vi "Stimulus trigger logic.vi"(7 "Abort triggers":bool, 8 "Unmodified signal values":T2, 9 "Stimulus Trigger Setup":T1={"Trigger period in live protocols (80MHz Cycles)"=80000000, "Pulse width in live protocols (80MHz Cycles)"=40000000, "Enable stimulus in live protocols"=FALSE, "Trigger delay in funct. protocols (80MHz Cycles)"=0, "Pulse width in funct. protocols (80MHz Cycles)"=400000, "Enable stimulus in funct. protocols"=FALSE}, 10 "live_scan":bool, 11 "Imaging Protocol":T3=enum."Live Imaging") -> (1 "Stimulus trigger":bool)   [LabVIEW 2020]
uses:
  <vilib>/eio/EIONode/EIONode.xnode
  <vilib>/rvi/eio/common/nirviEmuTemplateMethod_errors.vi
  Typedefs/Imaging Protocols enum.ctl
  FPGA Typedefs/PXI Trigger lines value cluster.ctl
  FPGA Typedefs/Stimulus trigger delays cluster.ctl
panel:
  # "Limited to 53.5 sec (if U32)"
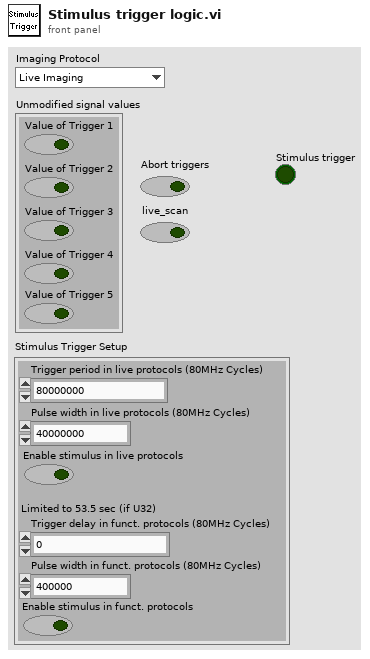
[diagram p1: front panel]
types:
  T1 = typedef "Stimulus trigger delays cluster.ctl" = cluster{"Trigger period in live protocols (80MHz Cycles)":u32, "Pulse width in live protocols (80MHz Cycles)":u32, "Enable stimulus in live protocols":bool, "Trigger delay in funct. protocols (80MHz Cycles)":u32, "Pulse width in funct. protocols (80MHz Cycles)":u32, "Enable stimulus in funct. protocols":bool}
  T2 = typedef "PXI Trigger lines value cluster.ctl" = cluster{"Value of Trigger 1":bool, "Value of Trigger 2":bool, "Value of Trigger 3":bool, "Value of Trigger 4":bool, "Value of Trigger 5":bool}
  T3 = typedef "Imaging Protocols enum.ctl" = enum16{"AOL Z-Stack", "Motor Z Stack", "Functional Acquisition", "Single Plane Acquisition", "Volume Acquisition", "Live Imaging", "Live Plane Imaging", "Live Volume Imaging"}
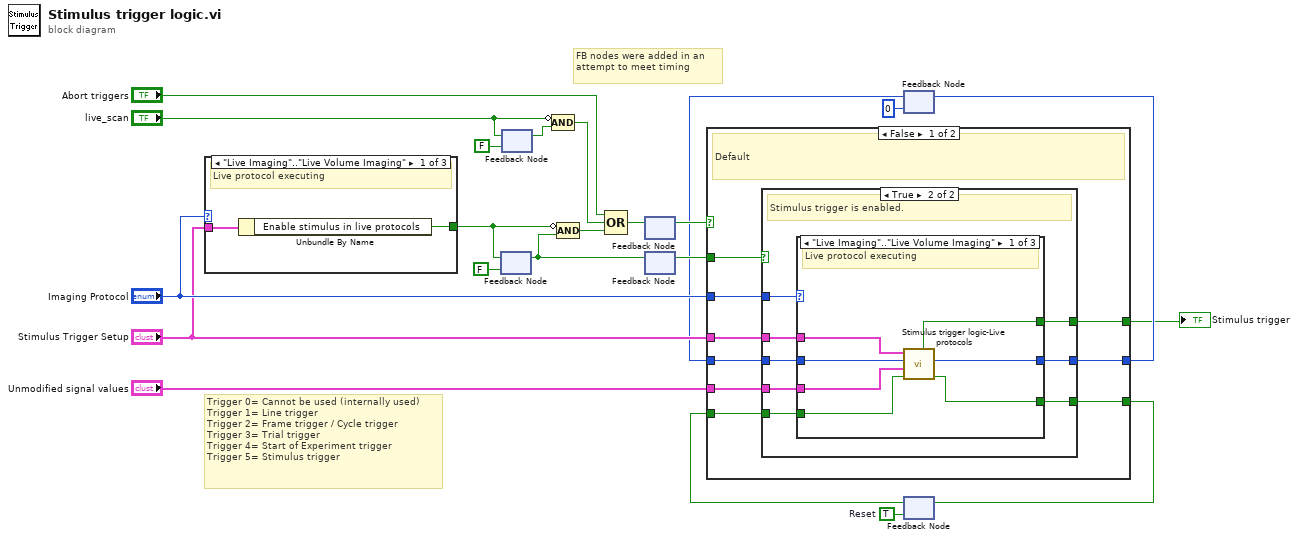
[diagram p0: block diagram]
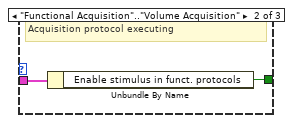
[diagram p2: hidden frame]
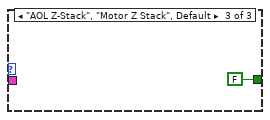
[diagram p3: hidden frame]
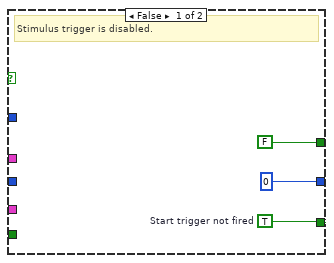
[diagram p4: hidden frame]
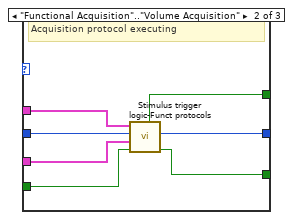
[diagram p5: hidden frame]
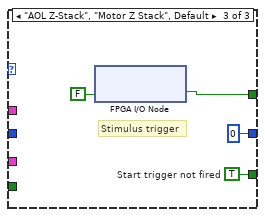
[diagram p6: hidden frame]
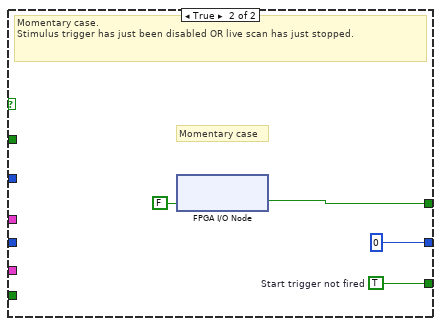
[diagram p7: hidden frame]
diagram:
  w16 = TRUE  # Reset
  # "FB nodes were added in an attempt to meet timing"
  # "Trigger 0= Cannot be used (internally used)\nTrigger 1= Line trigger\nTrigger 2= Frame trigger / Cycle trigger\nTrigger 3= Trial trigger\nTrigger 4= Start of Experiment trigger\nTrigger 5= Stimulus trigger"
  n1 = case shown="\"Live Imaging\"..\"Live Volume Imaging\"" "Imaging Protocol" {
    tunnel: "Stimulus Trigger Setup" -> [w24 w26 _]
    tunnel: [w23 w25 FALSE ("Enable stimulus in live protocols")] -> w12
    frame "Live Imaging".."Live Volume Imaging" {
      # "Live protocol executing"
      n2 = Unbundle By Name(w24) -> ("Enable stimulus in live protocols"=w23:bool)
    }
    frame "Functional Acquisition".."Volume Acquisition" {
      # "Acquisition protocol executing"
      n3 = Unbundle By Name(w26) -> ("Enable stimulus in funct. protocols"=w25:bool)
    }
    frame "AOL Z-Stack", "Motor Z Stack", Default {
    }
  }
  n4 = feedback #1(FALSE ("Trigger 1")) -> (w21:bool)
  n5 = feedback-in #1(w12) -> ()
  n6 = feedback #2(FALSE ("Trigger 1")) -> (w10:bool)
  n7 = feedback-in #2("live_scan") -> ()
  n8 = Compound Arithmetic op=AND(invert "live_scan", w10) -> (w8:bool)
  n9 = Compound Arithmetic op=AND(invert w12, w21) -> (w7:bool)
  n10 = Compound Arithmetic op=OR("Abort triggers", w8, w7) -> (w6:bool)
  n11 = feedback-in #3(w6) -> ()
  n12 = feedback #3() -> (w4:bool)  [unwired: 1 in]
  n13 = feedback-in #4(w21) -> ()
  n14 = feedback #4() -> (w5:bool)  [unwired: 1 in]
  n15 = feedback #5(u32 0 ("Tick Count(Ticks) out")) -> (w2:u32)
  n16 = feedback #6(w16) -> (w3:bool)
  n17 = case shown="False" w4 {
    tunnel: "Imaging Protocol" -> [w36 _]
    tunnel: w5 -> [w35 _]
    tunnel: "Unmodified signal values" -> [w34 _]
    tunnel: "Stimulus Trigger Setup" -> [w33 _]
    tunnel: [w32 w67] -> w18
    tunnel: w3 -> [w31 _]
    tunnel: [w30 u32 0 ("Tick Count(Ticks) out")] -> w19
    tunnel: w2 -> [w29 _]
    tunnel: [w28 w65] -> w15
    frame False {
      # "Default"
      n18 = case shown="True" w35 {
        tunnel: w36 -> [_ w47]
        tunnel: w34 -> [_ w46]
        tunnel: w33 -> [_ w45]
        tunnel: [w39 w41] -> w32
        tunnel: w31 -> [_ w44]
        tunnel: [u32 0 ("Tick Count(Ticks) out") w43] -> w30
        tunnel: w29 -> [_ w42]
        tunnel: [FALSE ("PXI_Trig0") w40] -> w28
        frame False {
          w39 = TRUE  # Start trigger not fired
          # "Stimulus trigger is disabled."
        }
        frame True {
          # "Stimulus trigger is enabled."
          n19 = case shown="\"Live Imaging\"..\"Live Volume Imaging\"" w47 {
            tunnel: w46 -> [w54 w61 _]
            tunnel: w45 -> [w52 w59 _]
            tunnel: w44 -> [w50 w57 _]
            tunnel: [w49 w56 u32 0 ("Tick Count(Ticks) out")] -> w43
            tunnel: w42 -> [w53 w60 _]
            tunnel: [w51 w58 w63] -> w41
            tunnel: [w48 w55 w62] -> w40
            frame "Live Imaging".."Live Volume Imaging" {
              # "Live protocol executing"
              n20 = call "Stimulus trigger logic-Live protocols.vi"("Start trigger not fired"=w50, "Trigger lines value"=w54, "Tick Count(Ticks) in"=w53, "Trigger delays"=w52) -> ("Start trigger not fired"=w51:bool, "Tick Count(Ticks) out"=w49:u32, "Output value"=w48:bool)  [unwired: 5 in]
            }
            frame "Functional Acquisition".."Volume Acquisition" {
              # "Acquisition protocol executing"
              n21 = call "Stimulus trigger logic-Funct protocols.vi"("Start trigger not fired"=w57, "Trigger lines value"=w61, "Tick Count(Ticks) in"=w60, "Stimulus Trigger Setup"=w59) -> ("Start trigger not fired"=w58:bool, "Tick Count(Ticks) out"=w56:u32, "Output value"=w55:bool)  [unwired: 5 in]
            }
            frame "AOL Z-Stack", "Motor Z Stack", Default {
              w62 = FALSE ("PXI_Trig0")
              w63 = TRUE  # Start trigger not fired
              # "Stimulus trigger"
              n22 = xnode "FPGA I/O Node"("PXI_Trig5"=w62) -> ()  [unwired: 1 in, 1 out]
            }
          }
        }
      }
    }
    frame True {
      w65 = FALSE ("PXI_Trig0")
      w67 = TRUE  # Start trigger not fired
      # "Momentary case"
      # "Momentary case.\nStimulus trigger has just been disabled OR live scan has just stopped."
      n23 = xnode "FPGA I/O Node"("PXI_Trig5"=w65) -> ()  [unwired: 1 in, 1 out]
    }
  }
  "Stimulus trigger" <- w15
  n24 = feedback-in #5(w19) -> ()
  n25 = feedback-in #6(w18) -> ()
